vi "Main.vi"() -> ()   [LabVIEW 2022 SP3]
uses:
  <vilib>/LabVIEW Interface for Arduino/Type Defs/Board Type.ctl
  <vilib>/LabVIEW Interface for Arduino/LabVIEW Interface for Arduino.lvlib
panel:
  in  "Total number of spins":i32=18
  out "Loop":i32
  in  "Iterations":i32=2
  in  "Output Filename":path=path "C:/Users/jerem/OneDrive/Desktop/Train_Data/run_n10_.lvm" caption="Filename"
  out "data":dynamicdata(graph)
  in  "Choo Choo?":bool
  out "time, s":dbl
  in  "Rate Hz":dbl=1000.0
  in  "Speed, m/s":sgl=1.0
  in  "FORWARD":bool=TRUE
  in  "VISA resource":refnum<visa-resource-name>="COM3"
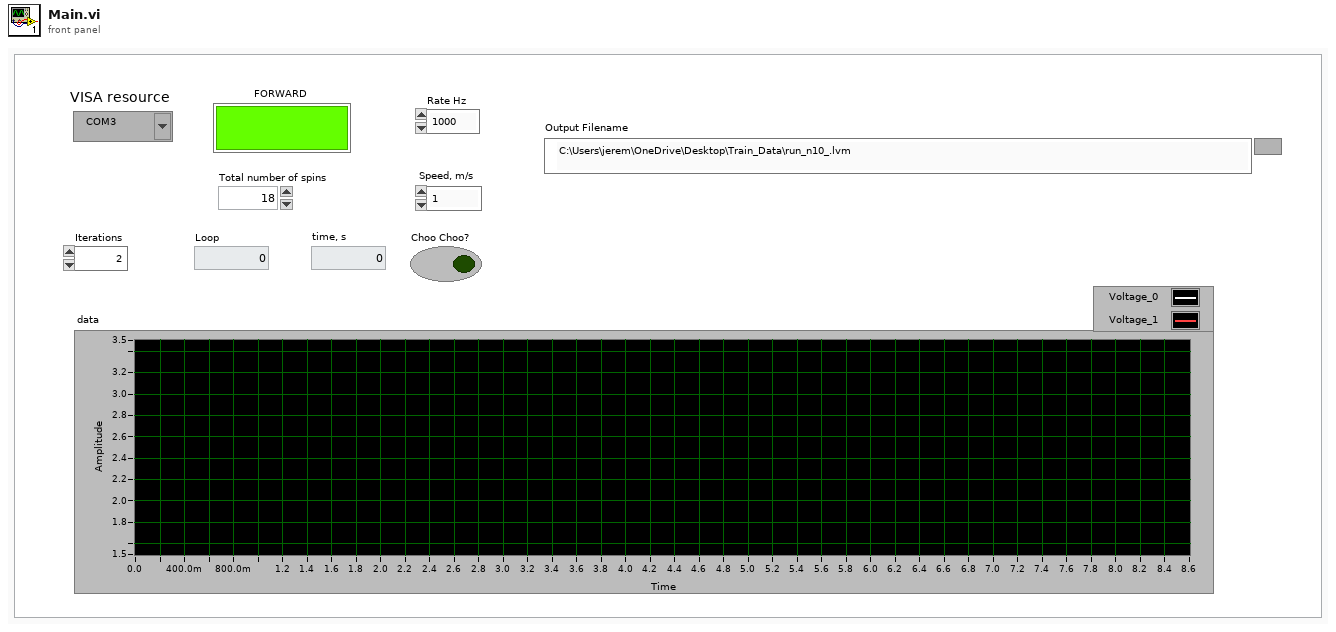
[diagram p1: front panel]
types:
  T1 = typedef "LabVIEW Interface for Arduino.lvlib/Board Type.ctl" = enum16{"Uno", "Dimuelanove w/Atmega 328", "Mega 2560"}
  T2 = typedef "LabVIEW Interface for Arduino.lvlib/Arduino Resource.ctl" = cluster{"VISA resource":refnum<visa-resource-name>, "Board Type":T1, "Connection Type":enum8{"USB / Serial"}, "Bytes Per Packet (15)":u8}
  T3 = typedef "Sound Output Task ID.ctl" = u32
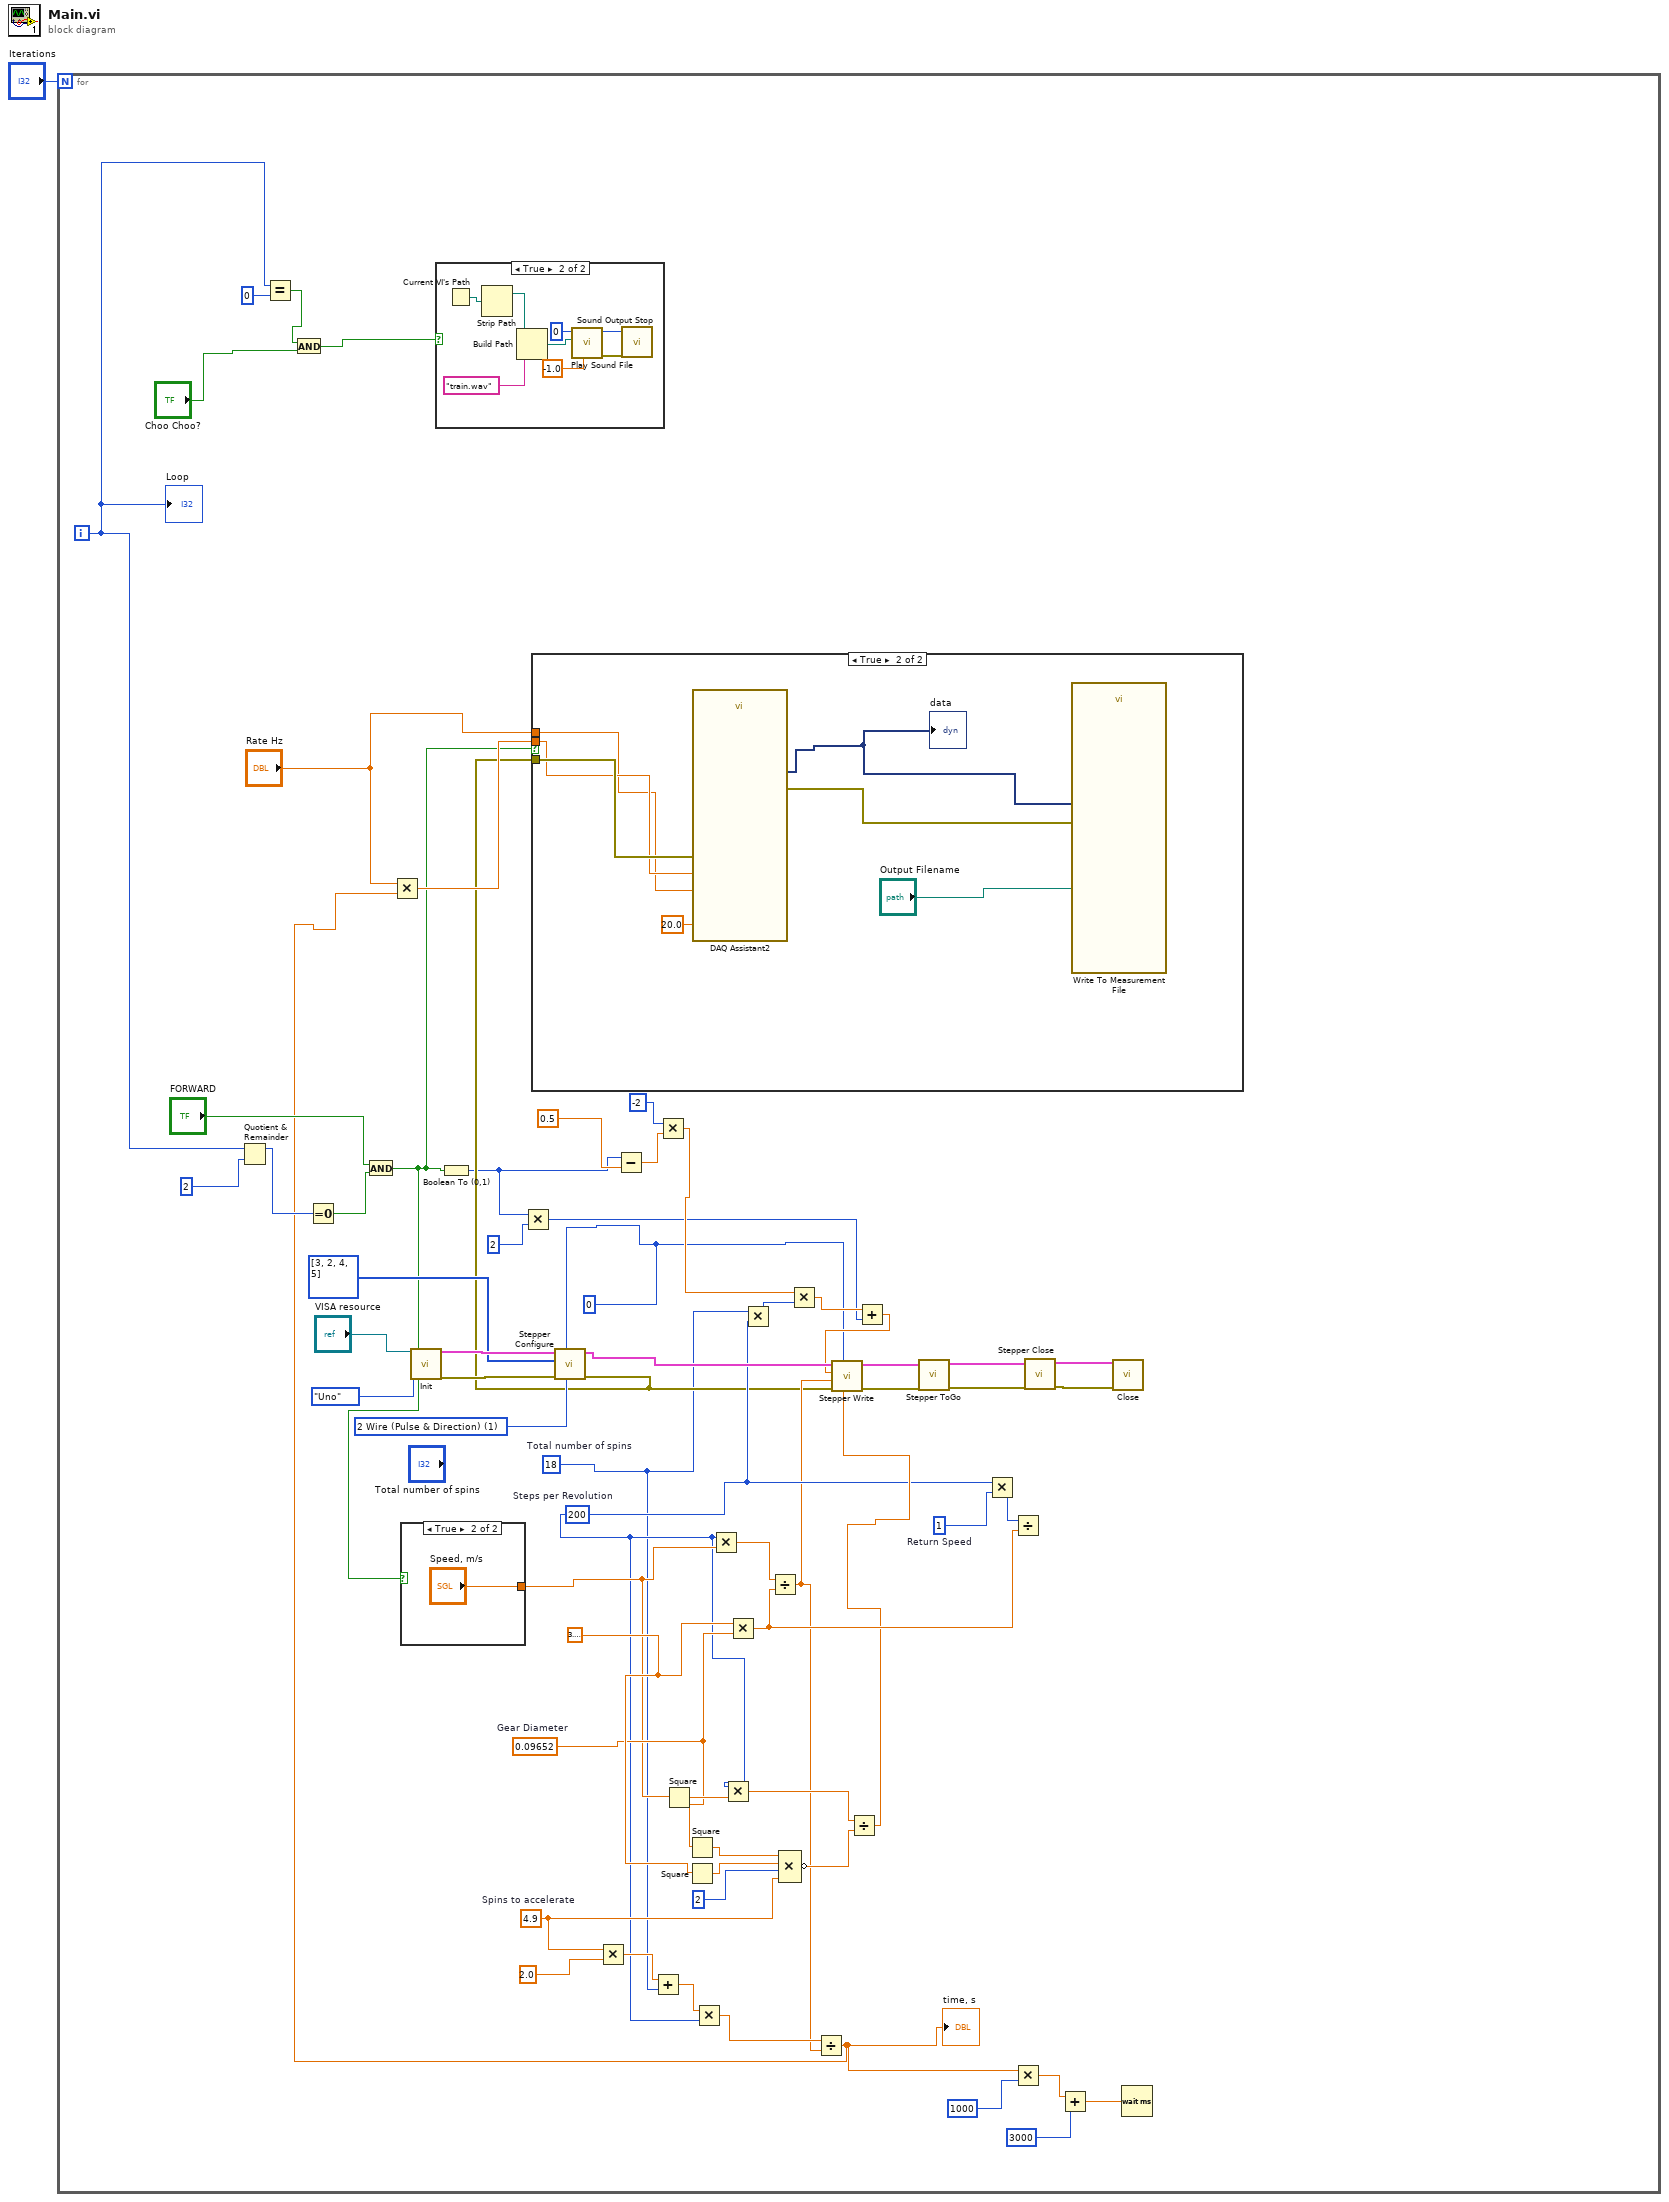
[diagram p0: block diagram]
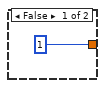
[diagram p3: hidden frame]
diagram:
  n1 = for {
    N: "Iterations" -> [_]
    i -> [w16]
    w24 = 18  # Total number of spins
    w51 = 1  # Return Speed
    w41 = 3.141592653589793
    w34 = 4.9  # Spins to accelerate
    w40 = 0.09652  # Gear Diameter
    w30 = i16 200  # Steps per Revolution
    w3 = u8 0 ("Stepper #")
    w61 = u8 1 items=["2 Wire (Pulse & Direction)"=1, "2 Wire"=2, "4 Wire"=4, "EasyDriver"=6, "AF Motor Shield (Stepper 1 & 2 Only)"=5] ("Control Method")
    n2 = Quotient & Remainder(x=w16, y=2) -> (x-y*floor(x/y)=w17:i32)  [unwired: 1 out]
    n3 = Equal?(x=w16, y=0) -> (x = y?=w20:bool)
    n4 = And(x=w20, y="Choo Choo?") -> (x .and. y?=w19:bool)
    n5 = Equal To 0?(x=w17) -> (x = 0?=w15:bool)
    n6 = And(x="FORWARD", y=w15) -> (x .and. y?=w13:bool)
    n7 = case shown="True" w13 {
      tunnel: [1 "Speed, m/s"] -> w39
      frame False {
      }
      frame True {
      }
    }
    n8 = call <vilib>:"Init.vi"("VISA resource"="VISA resource", "Board Type (Uno)"=Board_Type."Uno") -> ("Arduino Resource"=w65:T2, "error out"=w26:errorcluster)  [unwired: 16 in]
    n9 = case shown="True" w19 {
      frame False {
      }
      frame True {
        n10 = Current VI's Path() -> (path=w70:path)
        n11 = Strip Path(path=w70) -> (stripped path=w71:path)  [unwired: 1 out]
        n12 = Build Path(base path=w71, name or relative path="train.wav") -> (appended path=w73:path)
        n13 = call <vilib>:"Play Sound File.vi"("timeout (sec)"=-1.0, "path"=w73, "device ID"=u32 0) -> ("error out"=w66:errorcluster, "task ID"=w67:T3)  [unwired: 7 in]
        n14 = call <vilib>:"Sound Output Stop.vi"("error in (no error)"=w66, "task ID"=w67) -> ()  [unwired: 8 in, 2 out]
      }
    }
    n15 = Boolean To (0,1)(Boolean=w13) -> (0, 1=w7:i16)
    n16 = Multiply(x=w7, y=2) -> (x*y=w5:i32)
    n17 = call <vilib>:"Stepper Configure.vi"("Control Method"=w61, "Stepper #"=w3, "error in"=w26, "Stepper Pins"=u8[] [3, 2, 4, 5], "Arduino Resource"=w65) -> ("error out"=w25:errorcluster, "Arduino Resource Out"=w59:T2)  [unwired: 5 in]
    n18 = Multiply(x=w34, y=2.0) -> (x*y=w32:dbl)
    n19 = Subtract(x=w7, y=0.5) -> (x-y=w44:dbl)
    n20 = Add(x=w32, y=w24) -> (x+y=w31:dbl)
    n21 = Multiply(x=-2, y=w44) -> (x*y=w42:dbl)
    n22 = Square(x=w39) -> (x^2=w57:sgl)
    n23 = Square(x=w40) -> (x^2=w54:dbl)
    n24 = Square(x=w41) -> (x^2=w55:dbl)
    n25 = Multiply(x=w31, y=w30) -> (x*y=w29:dbl)
    n26 = Multiply(x=w30, y=w39) -> (x*y=w58:sgl)
    n27 = Multiply(x=w30, y=w57) -> (x*y=w53:sgl)
    n28 = Multiply(x=w41, y=w40) -> (x*y=w49:dbl)
    n29 = Multiply(x=w24, y=w30) -> (x*y=w47:i32)
    n30 = Divide(x=w58, y=w49) -> (x/y=w28:dbl)
    n31 = Compound Arithmetic op=MULTIPLY(w54, w55, 2, w34) -> (invert w52:dbl)
    n32 = Multiply(x=w42, y=w47) -> (x*y=w6:dbl)
    n33 = Divide(x=w29, y=w28) -> (x/y=w2:dbl)
    "time, s" <- w2
    n34 = Multiply(x="Rate Hz", y=w2) -> (x*y=w27:dbl)
    n35 = case shown="True" w13 {
      tunnel: "Rate Hz" -> [_ w79]
      tunnel: w27 -> [_ w80]
      tunnel: w25 -> [_ w81]
      frame False {
      }
      frame True {
        n36 = call "DAQ Assistant2"("rate"=w79, "number of samples"=w80, "timeout (s)"=20.0, "error in"=w81) -> ("data"=w77:dynamicdata, "error out"=w78:errorcluster)  [unwired: 12 in, 2 out]
        "data" <- w77
        n37 = call "Write To Measurement File"("Signals"=w77, "error in (no error)"=w78, "Filename"="Output Filename") -> ()  [unwired: 14 in, 3 out]
      }
    }
    n38 = Divide(x=w53, y=w52) -> (x/y=w48:dbl)
    n39 = Add(x=w6, y=w5) -> (x+y=w4:dbl)
    n40 = call <vilib>:"Stepper Write.vi"("Set Acceleration (0 to disable)"=w48, "Stepper #"=w3, "error in"=w25, "Set Speed (Steps per Second)"=w28, "# of Steps to Move"=w4, "Arduino Resource"=w59) -> ("error out"=w37:errorcluster, "Arduino Resource Out"=w38:T2)  [unwired: 4 in]
    n41 = call <vilib>:"Stepper ToGo.vi"("error in"=w37, "Arduino Resource"=w38) -> ("error out"=w36:errorcluster, "Arduino Resource Out"=w35:T2)  [unwired: 6 in, 2 out]
    n42 = Multiply(x=w30, y=w51) -> (x*y=w50:i32)
    n43 = Divide(x=w50, y=w49) -> ()  [unwired: 1 out]
    n44 = Multiply(x=w2, y=1000) -> (x*y=w11:dbl)
    n45 = call <vilib>:"Stepper Close.vi"("error in"=w36, "Arduino Resource"=w35) -> ("error out"=w62:errorcluster, "Arduino Resource Out"=w63:T2)  [unwired: 8 in]
    n46 = Add(x=w11, y=3000) -> (x+y=w9:dbl)
    n47 = call <vilib>:"Close.vi"("Arduino Resource"=w63, "error in"=w62) -> ()  [unwired: 13 in, 1 out]
    n48 = Wait (ms)(milliseconds to wait=w9) -> ()  [unwired: 1 out]
    "Loop" <- w16
  }
